vi "SERIAL_CalculateChecksum.vi"(2 "error in":errorcluster, 3 "Content":string) -> (0 "error out":errorcluster, 1 "Teminated Content":string)   [LabVIEW 2014, in "navX-MXP IMU.lvlib"]
uses:
  navX-MXP IMU.lvlib
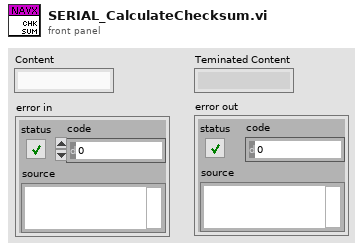
[diagram p1: front panel]
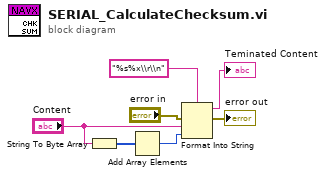
[diagram p0: block diagram]
diagram:
  n1 = String To Byte Array(string="Content") -> (unsigned byte array=w2:u8[])
  n2 = Add Array Elements(numeric array=w2) -> (sum=w1:u8)
  n3 = Format Into String(format string="%s%x\\r\\n" ("initial string"), error in="error in", "Content", w1) -> (resulting string=→"Teminated Content":string, error out=→"error out":errorcluster)  [unwired: 1 in]
